vi "Actor Core.vi"(8 "error in":errorcluster caption="entrée d'erreur", 11 "Cooler Panel in":refnum<class "Cooler Panel.lvclass"> caption="Acteur en entrée") -> (0 "error out":errorcluster caption="sortie d'erreur", 3 "Actor out":refnum<class "Actor.lvclass"> caption="Acteur en sortie")   [LabVIEW 2015, in "Cooler UI.lvlib" / "Cooler Panel.lvclass"]
doc: "(<B>Nom de fichier</B> : Actor Framework.lvlib:Actor.lvclass:Actor Core.vi)\n\nReçoit les messages destinés à l'acteur, y réagit et initialise toute gestion d'erreur susceptible de fermer l'acteur.\n\nLes classes descendantes peuvent redéfinir ce VI pour ajouter des tâches parallèles que l'acteur exécute tout en traitant les messages. Les redéfinitions utilisent le nœud Appeler la méthode parente."
uses:
  Cooler Panel.lvclass
  <vilib>/ActorFramework/Actor/Actor.lvclass
  <vilib>/ActorFramework/Actor/Actor.lvclass/Actor.ctl
  <vilib>/ActorFramework/Message Enqueuer/Message Enqueuer.lvclass/Message Enqueuer.ctl
  Cooler UI with Events/Cooler UI with Events.lvclass/Cooler UI with Events.ctl
  Cooler UI with Events Messages/Message Change Desired Temperature/Message Change Desired Temperature.lvclass/Message Change Desired Temperature.ctl
  <vilib>/ActorFramework/Message Enqueuer/Init from Existing Queue.vi
  <vilib>/ActorFramework/Message Enqueuer/Enqueue.vi
  <vilib>/ActorFramework/Message Priority Queue/Priority Enqueue.vi
  Cooler UI with Events/Cooler UI with Events.lvclass
  <vilib>/ActorFramework/Message Enqueuer/Message Enqueuer.lvclass
  Cooler UI with Events Messages/Message Change Desired Temperature/Message Change Desired Temperature.lvclass
panel:
  out "Pump":bool
  out "Temperature":dbl(slide) scale=0.0..120.0
  out "Fan A":bool
  out "Fan B":bool
  out "Fault A":bool
  out "Fault B":bool
  in  "Desired Temperature":dbl=75.0
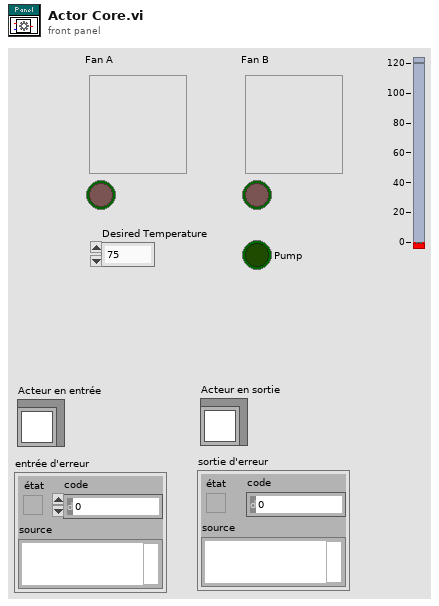
[diagram p1: front panel]
types:
  T1 = enum32{"Invalid", "Standard", "Closed", "Hidden", "Minimized", "Maximized"}
  T2 = typedef "Cooler UI.lvlib/Cooler UI with Events.lvclass/Events.ctl" = cluster{"Fan Status":refnum<user-event>, "Temperature":refnum<user-event>, "Pump":refnum<user-event>}
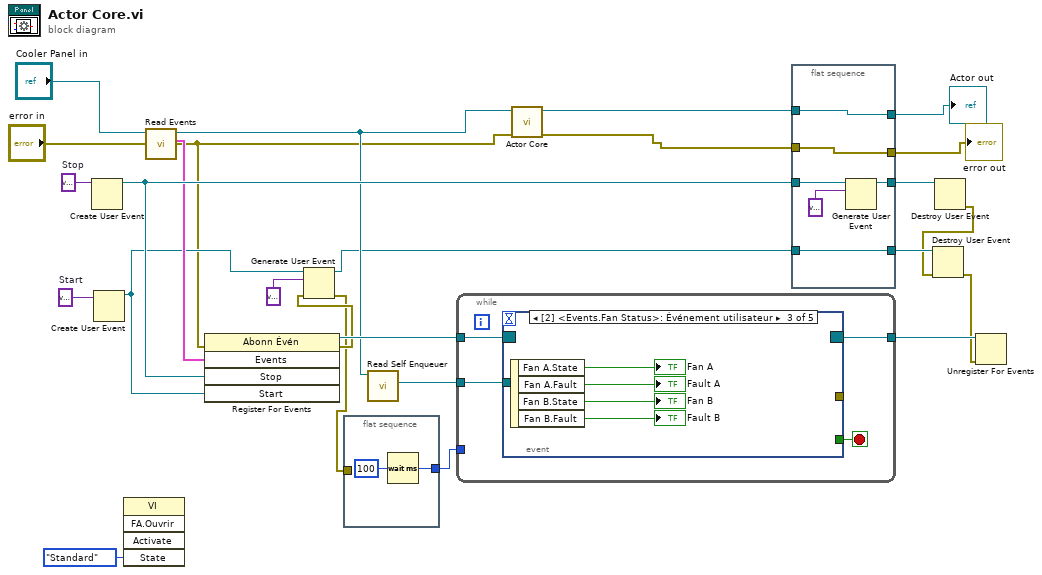
[diagram p0: block diagram]
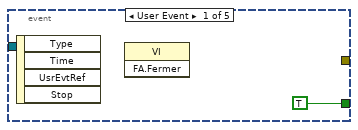
[diagram p2: hidden frame]
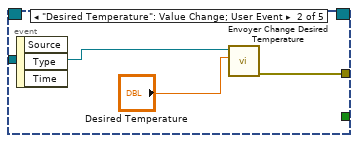
[diagram p3: hidden frame]
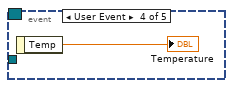
[diagram p4: hidden frame]
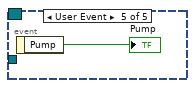
[diagram p5: hidden frame]
diagram:
  w11 = variant  # Start
  w22 = variant  # Stop
  n1 = Create User Event(user event datatype=w22) -> (user event=w20:refnum<user-event>)  [unwired: 1 in, 1 out]
  n2 = Create User Event(user event datatype=w11) -> (user event=w6:refnum<user-event>)  [unwired: 1 in, 1 out]
  n3 = invoke class="VI" method="FA.Ouvrir"("State"=T1."Standard") -> ()  [unwired: 4 in, 5 out]
  n4 = call "Read Events.vi"("Cooler UI with Events in"="Cooler Panel in") -> ("Events"=w19:T2, "Cooler UI with Events out"=w16:refnum<class "Cooler Panel.lvclass">)  [unwired: 9 in]
  n5 = register-events(error in="error in", w19, w20, w6) -> (reference out=w21:refnum<event-registration>, error out=w4:errorcluster)  [unwired: 1 in]
  n6 = Generate User Event(user event=w6, event data cluster=variant ("Stop"), error in=w4) -> (user event out=w5:refnum<user-event>, error out=w2:errorcluster)  [unwired: 1 in]
  n7 = flat-sequence {
    tunnel: w2 -> [_]
    tunnel: [w26] -> w1
    frame #0 {
      n8 = Wait (ms)(milliseconds to wait=u32 100 ("attente (ms)")) -> (millisecond timer value=w26:u32)
    }
  }
  n9 = call <vilib>:"Read Self Enqueuer.vi"("Actor"=w16) -> ("Self Enqueuer"=w18:refnum<class "Message Enqueuer.lvclass">)  [unwired: 10 in]
  n10 = while {
    tunnel: w21 -> [w31]
    tunnel: [w30] -> w23
    tunnel: w18 -> [w28]
    tunnel: w1 -> [_]
    stop <- w29 stop-if-true
    n11 = event shown="[2] <Events.Fan Status>: Événement utilisateur" {
      selector: w31 -> [_ _ _ _ _]
      dyn-events: [_ _ _ _ _] -> w30
      timeout: _ -> [_ _ _ _ _]
      tunnel: [TRUE _ _ _ _] -> w29
      tunnel: w28 -> [_ w34 _ _ _]
      tunnel: [_ w33 _ _ _] -> _
      event User Event {
        n12 = event-data() -> ()  [unwired: 1 in, 4 out]
        n13 = invoke class="VI" method="FA.Fermer"() -> ()  [unwired: 3 in, 3 out]
      }
      event "Desired Temperature": Value Change; User Event {
        n14 = event-data() -> ()  [unwired: 1 in, 3 out]
        n15 = call "Envoyer Change Desired Temperature.vi"("Desired Temperature"="Desired Temperature", "Message Enqueuer"=w34) -> ("error out"=w33:errorcluster)  [unwired: 8 in, 1 out]
      }
      event User Event {
        n16 = event-data() -> ("Fan A.State"=→"Fan A":bool, "Fan A.Fault"=→"Fault A":bool, "Fan B.State"=→"Fan B":bool, "Fan B.Fault"=→"Fault B":bool)  [unwired: 1 in]
      }
      event User Event {
        n17 = event-data() -> ("Temp"=→"Temperature":dbl)  [unwired: 1 in]
      }
      event User Event {
        n18 = event-data() -> ("Pump"=→"Pump":bool)  [unwired: 1 in]
      }
    }
  }
  n19 = call-parent "Actor Core.vi"("error in"="error in", "Actor in"=w16) -> ("error out"=w12:errorcluster, "Actor out"=w14:refnum<class "Actor.lvclass">)  [unwired: 8 in]
  n20 = flat-sequence {
    tunnel: [w47] -> w24
    tunnel: w20 -> [w46]
    tunnel: [w44] -> w15
    tunnel: w14 -> [w44]
    tunnel: [w43] -> w13
    tunnel: w12 -> [w43]
    tunnel: [w42] -> w10
    tunnel: w5 -> [w42]
    frame #0 {
      n21 = Generate User Event(user event=w46, event data cluster=variant ("Stop")) -> (user event out=w47:refnum<user-event>)  [unwired: 2 in, 1 out]
    }
  }
  n22 = Destroy User Event(user event=w24) -> (error out=w9:errorcluster)  [unwired: 1 in]
  n23 = Destroy User Event(user event=w10, error in=w9) -> (error out=w8:errorcluster)
  n24 = Unregister For Events(event registration refnum=w23, error in=w8) -> ()  [unwired: 1 out]
  "error out" <- w13
  "Actor out" <- w15
